vi "Input.vi"() -> ()   [LabVIEW 2011]
uses:
  Globals/Global IO.vi
panel:
  out "DI":bool[](array[boolean])
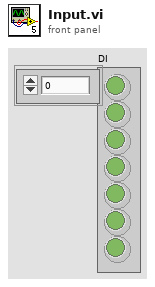
[diagram p1: front panel]
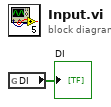
[diagram p0: block diagram]
diagram:
  n1 = global read "Global IO.vi" "DI"() -> (→"DI":bool[])
